vi "valuesToCSV.vi"(11 "number":dbl[](array[numeric])) -> (3 "concatenated values":string)   [LabVIEW 2012]
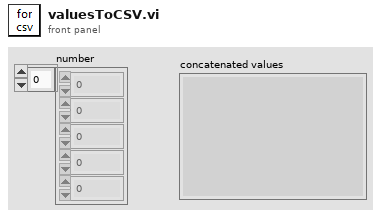
[diagram p1: front panel]
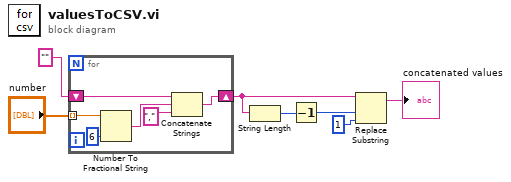
[diagram p0: block diagram]
diagram:
  n1 = for {
    tunnel: "number" -> [w13] mode=indexing
    shift-right: [w12] -> w3
    shift-left: "" -> [w11]
    n2 = Number To Fractional String(number=w13, precision (6)=i16 6) -> (F-format string=w10:string)  [unwired: 2 in]
    n3 = Concatenate Strings(w11, w10, "," ("string")) -> (w12:string)
  }
  n4 = String Length(string=w3) -> (length=w2:i32)
  n5 = Decrement(x=w2) -> (x-1=w1:i32)
  n6 = Replace Substring(2:1 ("length (len. of substring)"), 3:w1, 5:w3) -> (1:→"concatenated values":string)  [unwired: 1 in, 1 out]
